vi "FingerThreshold.vi"(2 "Threshold":dbl, 3 "task/channels in":refnum<k21>) -> (0 "VoltageCluster":cluster{"Index":dbl, "Middle":dbl, "Ring":dbl}, 1 "StatusCluster":T1)   [LabVIEW 2011]
uses:
  <vilib>/DAQmx/read.llb/DAQmx Read (Analog 1D DBL NChan 1Samp).vi
  <vilib>/DAQmx/miscellaneous.llb/DAQmx Fill In Error Info.vi
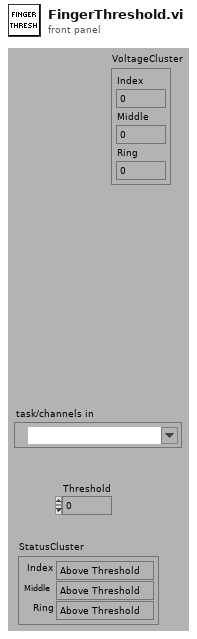
[diagram p1: front panel]
types:
  T1 = cluster{"Index":enum16{"Above Threshold", "Below Threshold"}, "Middle":enum16{"Above Threshold", "Below Threshold"}, "Ring":enum16{"Above Threshold", "Below Threshold"}}
  T2 = cluster{"data[0]":dbl, "data[1]":dbl, "data[2]":dbl}
  T3 = cluster{"[0]":enum16{"Above Threshold", "Below Threshold"}, "[1]":enum16{"Above Threshold", "Below Threshold"}, "[2]":enum16{"Above Threshold", "Below Threshold"}}
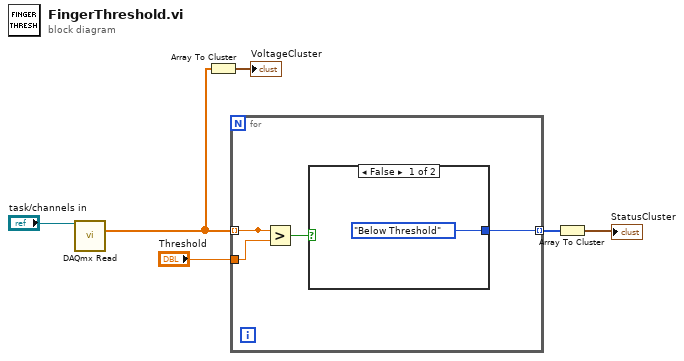
[diagram p0: block diagram]
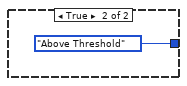
[diagram p2: hidden frame]
diagram:
  n1 = call-poly <vilib>:"DAQmx Read.vi"("task/channels in"="task/channels in") -> ("data"=w1:dbl[])  [unwired: 12 in, 2 out]
  n2 = Array To Cluster(array=w1) -> (cluster=→"VoltageCluster":T2)
  n3 = for {
    tunnel: [w10] -> _ mode=indexing
    tunnel: w1 -> [w10] mode=indexing
    tunnel: "Threshold" -> [w9]
    tunnel: [w7] -> w4 mode=indexing
    n4 = Greater?(x=w10, y=w9) -> (0:w8:bool)
    n5 = case shown="False" w8 {
      tunnel: [enum16{"Above Threshold", "Below Threshold"}."Below Threshold" ("Index") enum16{"Above Threshold", "Below Threshold"}."Above Threshold" ("Index")] -> w7
      frame False {
      }
      frame True {
      }
    }
  }
  n6 = Array To Cluster(array=w4) -> (cluster=→"StatusCluster":T3)
